vi "Configure Websockets MQTT Connection.vi"(5 "WSConnection in":refnum<class "WebsocketsConnection.lvclass">, 6 "timeout (5000 ms)":i32=5000, 8 "error in (no error)":errorcluster, 9 "path":string="/", 10 "remote port (80)":u16=80, 11 "address (localhost)":string="localhost") -> (0 "error out":errorcluster, 3 "WSConnection":refnum<class "WebsocketsConnection.lvclass">)   [LabVIEW 2013, in "MQTT_Websockets.lvlib" / "WebsocketsConnection.lvclass"]
uses:
  WebsocketsConnection.lvclass
  <vilib>/LabVIEW Open Source Project/Connection/Connection.Websockets/Connection.WS.lvclass
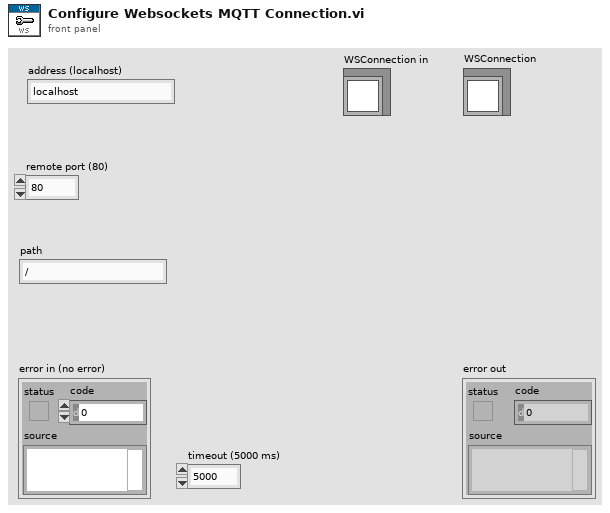
[diagram p1: front panel]
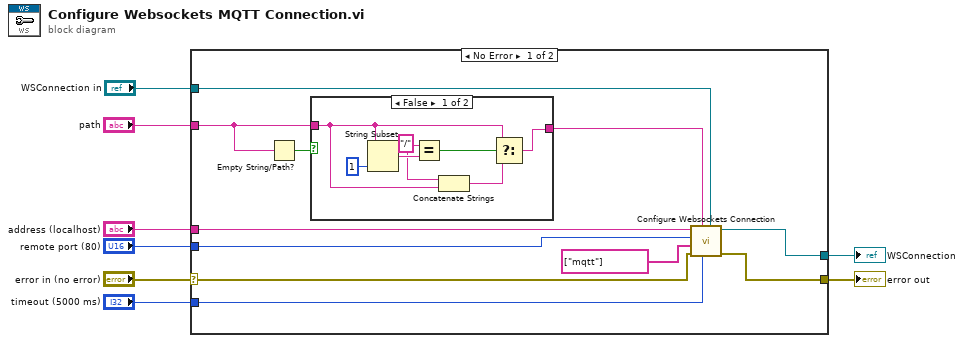
[diagram p0: block diagram]
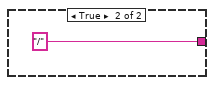
[diagram p2: hidden frame]
diagram:
  n1 = case shown="No Error" "error in (no error)" {
    selector: "error in (no error)" -> [w13 w29]
    tunnel: [w14 w29] -> w7
    tunnel: [w18 w28] -> w3
    tunnel: "address (localhost)" -> [w16 _]
    tunnel: "remote port (80)" -> [w17 _]
    tunnel: "timeout (5000 ms)" -> [w15 _]
    tunnel: "path" -> [w10 _]
    tunnel: "WSConnection in" -> [w19 w28]
    frame No Error {
      n2 = Empty String/Path?(string/path=w10) -> (empty?=w12:bool)
      n3 = case shown="False" w12 {
        tunnel: [w23 "/" ("path (/)")] -> w11
        tunnel: w10 -> [w21 _]
        frame False {
          w22 = "/" ("x")
          n4 = String Subset(string=w21, length (rest)=1 ("length (rest)")) -> (substring=w25:string)  [unwired: 1 in]
          n5 = Equal?(x=w22, y=w25) -> (x = y?=w24:bool)
          n6 = Concatenate Strings(w22, w21) -> (w20:string)
          n7 = Select(t=w21, s=w24, f=w20) -> (s? t:f=w23:string)
        }
        frame True {
        }
      }
      n8 = call <vilib>:"Configure Websockets Connection.vi"("Connection.Websockets"=w19, "timeout (5000ms)"=w15, "path (/)"=w11, "error in (no error)"=w13, "subProtocols"=string[] ["mqtt"], "remote port (80)"=w17, "address (localhost)"=w16) -> ("error out"=w14:errorcluster, "Connection.Websockets"=w18:refnum<class "WebsocketsConnection.lvclass">)  [unwired: 3 in]
    }
    frame Error {
    }
  }
  "error out" <- w7
  "WSConnection" <- w3
